vi "InitializeLog_HRI.vi"() -> (3 "refnum out":refnum<file>)   [LabVIEW 2018]
panel:
  in  "Format":string="=====================================================================================================================\nTIME       Time2(ms)             count             rawX                rawY               X                Y              Z( zoom)            Pause             Finish_late\n====================================================================================================================="
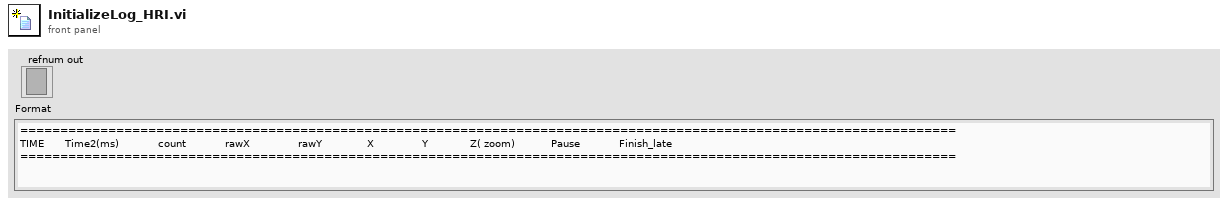
[diagram p1: front panel]
types:
  T1 = enum16{"open", "replace", "create", "open or create", "replace or create", "replace or create with confirmation"}
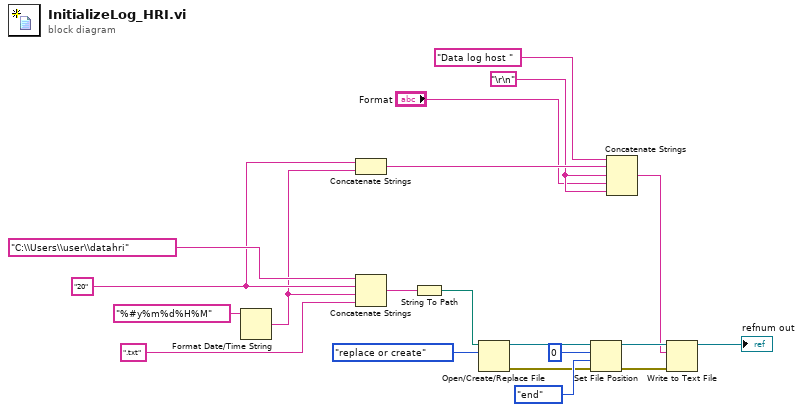
[diagram p0: block diagram]
diagram:
  w4 = "\r\n"
  w7 = "20" ("string")
  n1 = Format Date/Time String(time format string (%c)="%#y%m%d%H%M" ("string")) -> (date/time string=w6:string)  [unwired: 2 in]
  n2 = Concatenate Strings(w7, w6) -> (w5:string)
  n3 = Concatenate Strings("C:\\Users\\user\\datahri" ("string"), w7, w6, ".txt" ("string")) -> (w8:string)
  n4 = String To Path(string=w8) -> (path=w1:path)
  n5 = Open/Create/Replace File(file path (use dialog)=w1, operation (0:open)=T1."replace or create") -> (refnum out=w16:refnum<file>, error out=w12:errorcluster)  [unwired: 4 in, 1 out]
  n6 = Set File Position(offset (in bytes) (0)=i64 0, refnum=w16, from (0:start)=enum16{"start", "end", "current"}."end", error in=w12) -> (refnum out=w13:refnum<file>, error out=w11:errorcluster)
  n7 = Concatenate Strings("Data log host " ("string"), w5, w4, "Format", w4) -> (w10:string)
  n8 = Write to Text File(file (use dialog)=w13, text=w10, error in=w11) -> (refnum out=→"refnum out":refnum<file>)  [unwired: 1 in, 2 out]
